vi "ULx Write (Analog 1D Wfm NChan 1Samp).vi"(0 "task in":refnum<k24>, 1 "auto start":bool=TRUE, 7 "data":waveform(dbl)[](array[waveform]), 9 "timeout":dbl=10.0 format="%_4g", 11 "error in":errorcluster) -> (4 "task out":refnum<k24>, 10 "number of samples written per channel":u32, 15 "error out":errorcluster)   [LabVIEW 2020]
doc: "Writes a waveform that contains a single sample to each channel in a task that contains one or more analog output channels."
uses:
  C:/Users/William/Documents/LV 2020 builds/LeaktestDAQ/Source-v33/ULx_LV.dll
  ULx_LV.dll
panel:
  # "channel"
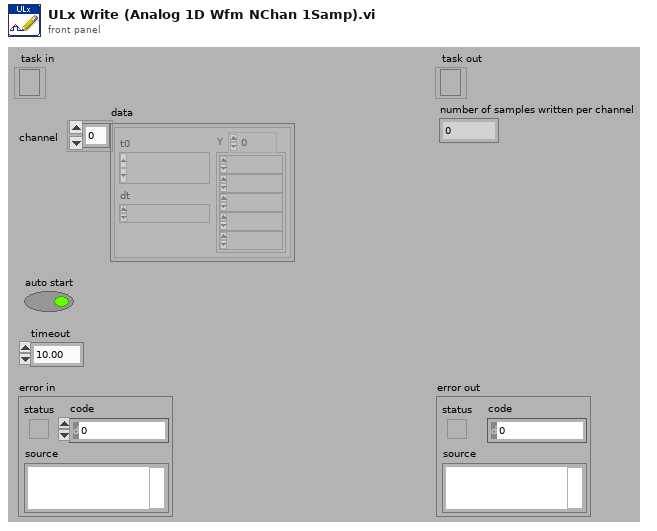
[diagram p1: front panel]
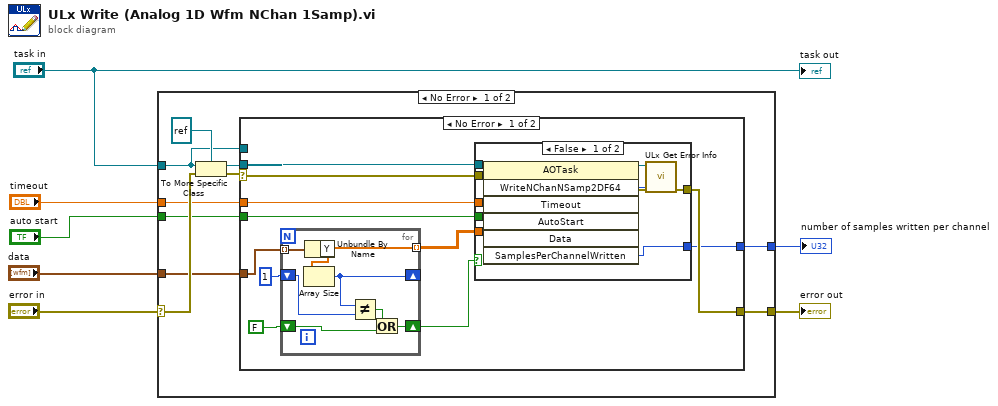
[diagram p0: block diagram]
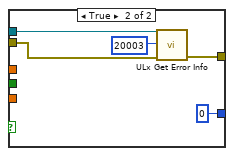
[diagram p2: hidden frame]
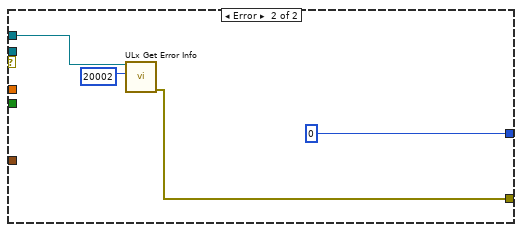
[diagram p3: hidden frame]
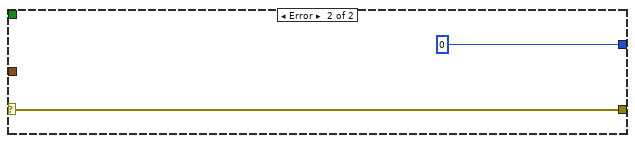
[diagram p4: hidden frame]
diagram:
  n1 = case shown="No Error" "error in" {
    selector: "error in" -> [w17 w56]
    tunnel: "task in" -> [w11 _]
    tunnel: "timeout" -> [w13 _]
    tunnel: [w12 w56] -> w5
    tunnel: "data" -> [w8 _]
    tunnel: "auto start" -> [w10 _]
    tunnel: [w9 0 ("SamplesPerChannelWritten")] -> w2
    frame No Error {
      n2 = To More Specific Class(target class=refnum<k24> refnum, reference=w11, error in=w17) -> (specific class reference=w14:refnum<k24>, error out=w15:errorcluster)
      n3 = case shown="No Error" w15 {
        selector: w15 -> [w27 _]
        tunnel: w14 -> [w28 _]
        tunnel: w13 -> [w24 _]
        tunnel: [w26 w53] -> w12
        tunnel: w11 -> [_ w52]
        tunnel: w10 -> [w23 _]
        tunnel: [w25 0 ("SamplesPerChannelWritten")] -> w9
        tunnel: w8 -> [w21 _]
        frame No Error {
          n4 = for {
            shift-right: [w49] -> _
            shift-left: 1 -> [w48]
            tunnel: [w50] -> w22 mode=indexing
            tunnel: w21 -> [w47] mode=indexing
            shift-right: [w46] -> w19
            shift-left: FALSE -> [w45]
            n5 = Unbundle By Name(w47) -> ("Y"=w50:dbl[])
            n6 = Array Size(array=w50) -> (size(s)=w49:i32)
            n7 = Not Equal?(x=w49, y=w48) -> (x != y?=w44:bool)
            n8 = Or(x=w44, y=w45) -> (x .or. y?=w46:bool)
          }
          n9 = case shown="False" w19 {
            tunnel: w28 -> [w38 w40]
            tunnel: w27 -> [w37 w39]
            tunnel: [w34 w43] -> w26
            tunnel: [w32 u32 0 ("SamplesPerChannelWritten")] -> w25
            tunnel: w24 -> [w31 _]
            tunnel: w23 -> [w30 _]
            tunnel: w22 -> [w29 _]
            frame False {
              n10 = invoke class="AOTask" method="WriteNChanNSamp2DF64"(reference=w38, error in=w37, "Timeout"=w31, "AutoStart"=w30, "Data"=w29) -> (reference out=w35:refnum<k24>, error out=w36:errorcluster, "WriteNChanNSamp2DF64"=w33:i32, "SamplesPerChannelWritten"=w32:u32)  [unwired: 2 in, 3 out]
              n11 = call "ULx Get Error Info.vi"("error in"=w36, "ErrorCode"=w33, "task in"=w35) -> ("error out"=w34:errorcluster)  [unwired: 8 in]
            }
            frame True {
              n12 = call "ULx Get Error Info.vi"("error in"=w39, "ErrorCode"=20003, "task in"=w40) -> ("error out"=w43:errorcluster)  [unwired: 8 in]
            }
          }
        }
        frame Error {
          n13 = call "ULx Get Error Info.vi"("ErrorCode"=20002, "task in"=w52) -> ("error out"=w53:errorcluster)  [unwired: 9 in]
        }
      }
    }
    frame Error {
    }
  }
  "error out" <- w5
  "number of samples written per channel" <- w2
  "task out" <- "task in"
